vi "ccc_Convert From Compatibility TagConfig.vi"(11 "old tag":T4) -> (3 "new tag":T1)   [LabVIEW 2010]
uses:
  ccc_TagConfiguration.ctl
  <vilib>/NI/Current Value Table/Compatibility/_SubVIs/TypeDefs/cvt_Data Types.ctl
  ccc_TagDirection.ctl
  Tag Configuration.ctl
  <vilib>/NI/Current Value Table/Type Defs/Data Types.ctl
  Tag Direction.ctl
  <vilib>/NI/Current Value Table/Current Value Table.lvlib
  NI_CCC.lvlib
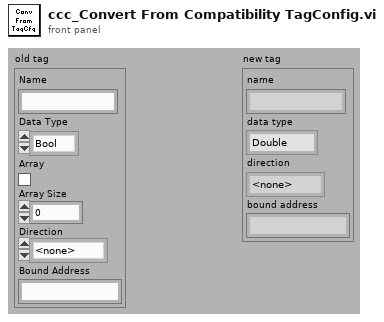
[diagram p1: front panel]
types:
  T1 = typedef "NI_CCC.lvlib/Tag Configuration.ctl" = cluster{"name":string, "data type":T2, "direction":T3, "bound address":string}
  T2 = typedef "Current Value Table.lvlib/Data Types.ctl" = enum16{"Double", "Single", "I64", "I32", "I16", "I8", "U64", "U32", "U16", "U8", "String", "Boolean", "Array of U8", "Array of U16", "Array of U32", "Array of U64", "Array of I64", "Array of I32", "Array of I16", "Array of I8", "Array of Double", "Array of Single", "Array of Boolean", "Array of String"}
  T3 = typedef "NI_CCC.lvlib/Tag Direction.ctl" = enum32{"<none>", "Read", "Write"}
  T4 = typedef "ccc_TagConfiguration.ctl" = cluster{"Name":string, "Data Type":T5, "Array":bool, "Array Size":u32, "Direction":T6, "Bound Address":string}
  T5 = typedef "cvt_Data Types.ctl" = enum16{"Bool", "U8", "I32", "Double", "String", "Enum"}
  T6 = typedef "ccc_TagDirection.ctl" = enum32{"<none>", "Read", "Write"}
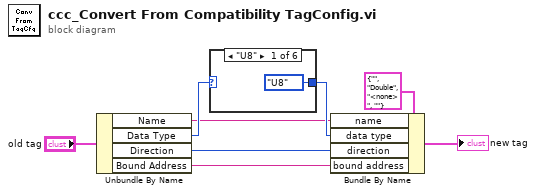
[diagram p0: block diagram]
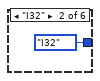
[diagram p2: hidden frame]
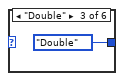
[diagram p3: hidden frame]
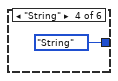
[diagram p4: hidden frame]
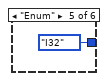
[diagram p5: hidden frame]
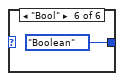
[diagram p6: hidden frame]
diagram:
  n1 = Unbundle By Name("old tag") -> ("Name"=w4:string, "Data Type"=w7:T5, "Direction"=w5:T6, "Bound Address"=w6:string)
  n2 = case shown="\"U8\"" w7 {
    tunnel: [Data_Types."U8" ("Data Type") Data_Types."I32" ("Data Type") Data_Types."Double" ("Data Type") Data_Types."String" ("Data Type") Data_Types."I32" ("Data Type") Data_Types."Boolean" ("Data Type")] -> w8
    frame "U8" {
    }
    frame "I32" {
    }
    frame "Double" {
    }
    frame "String" {
    }
    frame "Enum" {
    }
    frame "Bool" {
    }
  }
  n3 = Bundle By Name(cluster=T1 {"name"="", "data type"=enum."Double", "direction"=enum."<none>", "bound address"=""} ("HMI DataEngine Tag List"), "name"=w4, "data type"=w8, "direction"=w5, "bound address"=w6) -> (→"new tag":T1)
